vi "Allocate Single Block.vi"(8 "error in (no error)":errorcluster, 10 "size (bytes)":i32, 11 "GE 5565PIORC in":refnum<class "GE 5565PIORC.lvclass">) -> (0 "error out":errorcluster, 2 "Block Descriptor":T1 {"next descriptor ptr" format="%08x"; "data size" format="%08x"; "data ptr (upper)" format="%08x"; "data ptr (lower)" format="%08x"; "descriptor ptr (aligned)" format="%08x"; "descriptor size" format="%08x"; "descriptor ptr (VISA)" format="%08x"}, 3 "GE 5565PIORC out":refnum<class "GE 5565PIORC.lvclass">)   [LabVIEW 2016, in "GE 5565PIORC.lvclass"]
uses:
  GE 5565PIORC.lvclass
  Controls/DMA Block Descriptor.ctl
  GE 5565PIORC.lvclass/GE 5565PIORC.ctl
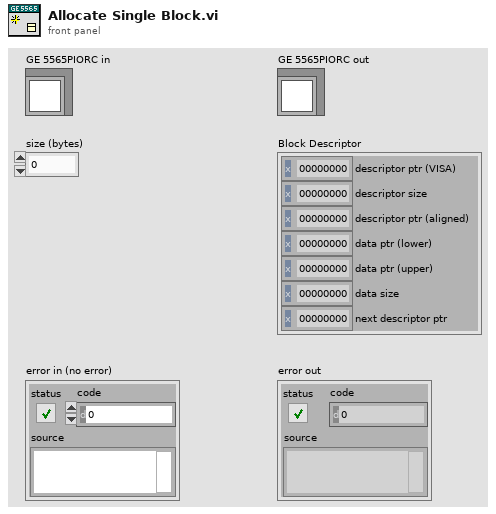
[diagram p1: front panel]
types:
  T1 = typedef "GE 5565PIORC.lvclass/DMA Block Descriptor.ctl" = cluster{"descriptor ptr (VISA)":u32, "descriptor size":u32, "descriptor ptr (aligned)":u32, "data ptr (lower)":u32, "data ptr (upper)":u32, "data size":u32, "next descriptor ptr":u32}
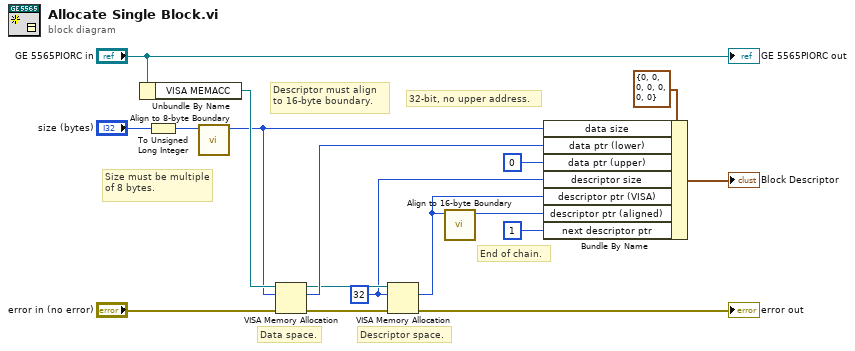
[diagram p0: block diagram]
diagram:
  w9 = u32 32 ("size")
  # "Descriptor must align to 16-byte boundary."
  # "Descriptor space."
  # "Data space."
  # "32-bit, no upper address."
  # "End of chain."
  # "Size must be multiple of 8 bytes."
  n1 = Unbundle By Name("GE 5565PIORC in") -> ("VISA MEMACC"=w4:refnum<visa-resource-name>)
  n2 = To Unsigned Long Integer(number="size (bytes)") -> (unsigned 32bit integer=w1:u32)
  n3 = call "Align to 8-byte Boundary.vi"("pointer"=w1) -> ("aligned pointer"=w3:u32)  [unwired: 10 in]
  n4 = VISA Memory Allocation(8:"error in (no error)", 10:w3, 11:w4) -> (0:w13:errorcluster, 2:w16:u32, 3:w12:refnum<visa-resource-name>)
  n5 = VISA Memory Allocation(8:w13, 10:w9, 11:w12) -> (0:→"error out":errorcluster, 2:w8:u32)  [unwired: 1 out]
  n6 = call "Align to 16-byte Boundary.vi"("pointer"=w8) -> ("aligned pointer"=w7:u32)  [unwired: 10 in]
  n7 = Bundle By Name(cluster=T1 {"descriptor ptr (VISA)"=0, "descriptor size"=0, "descriptor ptr (aligned)"=0, "data ptr (lower)"=0, "data ptr (upper)"=0, "data size"=0, "next descriptor ptr"=0} ("Block Descriptor"), "data size"=w3, "data ptr (lower)"=w16, "data ptr (upper)"=u32 0 ("next block pointer"), "descriptor size"=w9, "descriptor ptr (VISA)"=w8, "descriptor ptr (aligned)"=w7, "next descriptor ptr"=u32 1 ("next block pointer")) -> (→"Block Descriptor":T1)
  "GE 5565PIORC out" <- "GE 5565PIORC in"
